vi "Scales gradients.vi"(1 "Shifts, B":dbl[](array[numeric]) format="%.3f", 2 "Tau, t":dbl[](array[numeric]) format="%.3f") -> (0 "Scales, A":dbl[](array[numeric]) format="%.3f")   [LabVIEW 2022 SP3]
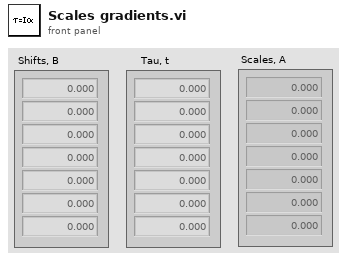
[diagram p1: front panel]
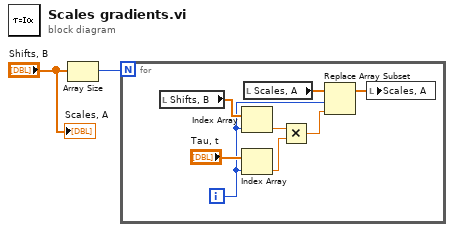
[diagram p0: block diagram]
diagram:
  n1 = Array Size(array="Shifts, B") -> (size(s)=w2:i32)
  n2 = for {
    N: w2 -> [_]
    i -> [w4]
    n3 = local read "Shifts, B"() -> (w9:dbl[])
    n4 = Index Array(array=w9, index=w4) -> (element=w8:dbl)
    n5 = Index Array(array="Tau, t", index=w4) -> (element=w7:dbl)
    n6 = local read "Scales, A"() -> (w6:dbl[])
    n7 = Multiply ("Multiply.vi")(x=w8, y=w7) -> (x*y=w3:dbl)
    n8 = Replace Array Subset(array=w6, new element=w3, index=w4) -> (w5:dbl[])
    n9 = local write "Scales, A"(w5) -> ()
  }
  "Scales, A" <- "Shifts, B"
